vi "LVClass_ModalCoef SetLegendrePrefs.vi"(0 "ModalCoef in":refnum<class "ModalCoef.lvclass">, 5 "LegendreModalPrefs":T1={"Number of coefficients"=32, "Filtered coefficients"=[], "RectangularProjectionPupilDimensions"={"Pupil center_sspp"={"X"=0.0, "Y"=0.0}, "Pupil halfsize_sspp"={"X"=0.0, "Y"=0.0}}}, 11 "error in (no error)":errorcluster) -> (4 "ModalCoef out":refnum<class "ModalCoef.lvclass">, 15 "error out":errorcluster)   [LabVIEW 2020, in "ModalCoef.lvclass"]
doc: "Set the Legendre preferences for modal phase reconstruction.\n\n--------------------------------------------------------------------------------\n\n<B>ComputePhaseSetIn </B> : ComputePhaseSet object.\n<B>ComputePhaseSetOut </B> : ComputePhaseSet object.\n<B>nb_coeffs_total </B> : Number of the Legendre coefficients used in the polynomial base.\n<B>nb_coeffs_to_filter </B> : Number of the Legendre coefficients to filter in the polynomial base.\n<B>coeffs_to_filter </B> : List of indices of the Legendre coefficients to filter in the polynomial base.\n<B>projection_pupil_center </B> : Center of the projection pupil, in number of subpupils.\n<B>projection_pupil_halfsize </B> : Projection pupil half size, in number of subpupils.\n<B>ErrorIn </B> : Error\n<B>ErrorOut </B> : Error\n\n--------------------------------------------------------------------------------"
uses:
  ModalCoef.lvclass
  LegendreModalPrefs.ctl
  LegendreProjectionPupilSetup.ctl
  Point2Df.ctl
  ModalCoef.lvclass/ModalCoef.ctl
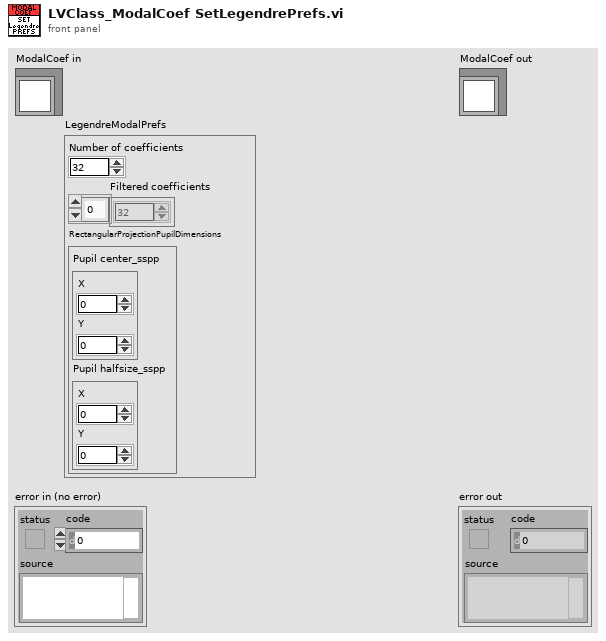
[diagram p1: front panel]
types:
  T1 = typedef "LegendreModalPrefs.ctl" = cluster{"Number of coefficients":u32, "Filtered coefficients":u32[], "RectangularProjectionPupilDimensions":T2}
  T2 = typedef "LegendreProjectionPupilSetup.ctl" = cluster{"Pupil center_sspp":T3, "Pupil halfsize_sspp":T3}
  T3 = typedef "Point2Df.ctl" = cluster{"X":sgl, "Y":sgl}
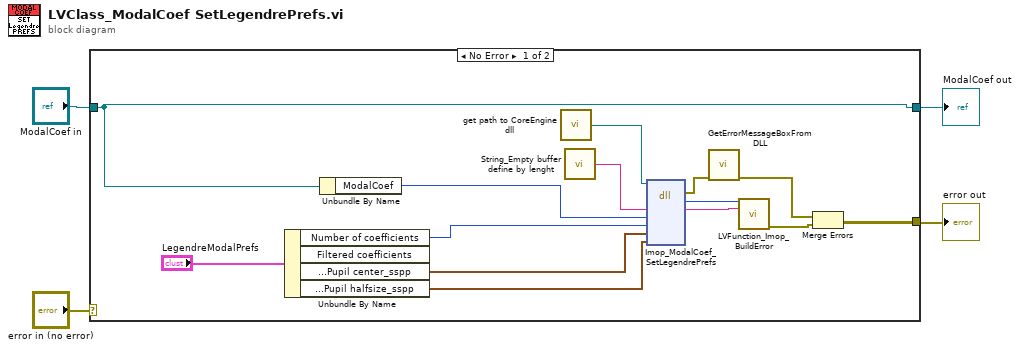
[diagram p0: block diagram]
diagram:
  n1 = case shown="No Error" "error in (no error)" {
    selector: "error in (no error)" -> [_ w20]
    tunnel: [w5 w20] -> w1
    tunnel: [w9 w19] -> w3
    tunnel: "ModalCoef in" -> [w9 w19]
    frame No Error {
      n2 = Unbundle By Name("LegendreModalPrefs") -> ("Number of coefficients"=w12:u32, "RectangularProjectionPupilDimensions.Pupil center_sspp"=w11:T3, "RectangularProjectionPupilDimensions.Pupil halfsize_sspp"=w10:T3)  [unwired: 1 out]
      n3 = Unbundle By Name(w9) -> ("ModalCoef"=w8:i32)
      n4 = call "get path to CoreEngine dll.vi"() -> ("path to c_interface_vc100.dll"=w15:path)  [unwired: 12 in, 3 out]
      n5 = call "String_Empty buffer define by lenght.vi"() -> ("Empty buffer"=w16:string)  [unwired: 1 in]
      n6 = dll-call lib="D:/2_trunk/Soft_haso/ImOpCoreEngine4_LV2011/DLLs/ImopEngine4_vc100.dll" fn="Imop_ModalCoef_SetLegendrePrefs"(path in=w15, "message"=w16, "objet"=w8, "numberOfCoefficient"=w12, "projection_pupil_center"=w11, "projection_pupil_size"=w10) -> (error out=w14:errorcluster, "return type"=w18:i32, "message"=w17:string)  [unwired: 6 in, 1 out]
      n7 = call "GetErrorMessageBoxFromDLL.vi"("error IN"=w14) -> ("error OUT"=w7:errorcluster)  [unwired: 10 in]
      n8 = call "LVFunction_Imop_BuildError.vi"("code"=w18, "String to Prepend to source (\"\")"=w17) -> ("error out"=w6:errorcluster)  [unwired: 13 in]
      n9 = Merge Errors(w7, w6) -> (w5:errorcluster)
    }
    frame Error {
    }
  }
  "error out" <- w1
  "ModalCoef out" <- w3
